vi "test Handle To Owned.vi"(8 "error in (no error)":errorcluster, 11 "TestCase in":refnum<class "Memory Manager Tests.lvclass">) -> (0 "error out":errorcluster, 3 "TestCase out":refnum<class "Memory Manager Tests.lvclass">)   [LabVIEW 2020, in "Memory Manager Tests.lvclass"]
uses:
  Memory Manager Tests.lvclass
  <vilib>/Utility/file.llb/Application Directory.vi
  <vilib>/Utility/libraryn.llb/Check if File or Folder Exists.vi
  <vilib>/addons/_JKI Toolkits/VI Tester/TestCase.llb/TestCase.lvclass
  C:/Program Files/National Instruments/LabVIEW 2024/vi.lib/addons/_JKI Toolkits/VI Tester/TestCase.llb/TestCase.lvclass
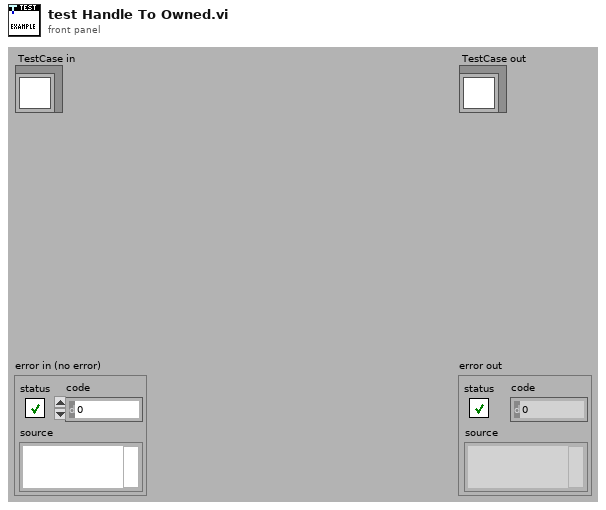
[diagram p1: front panel]
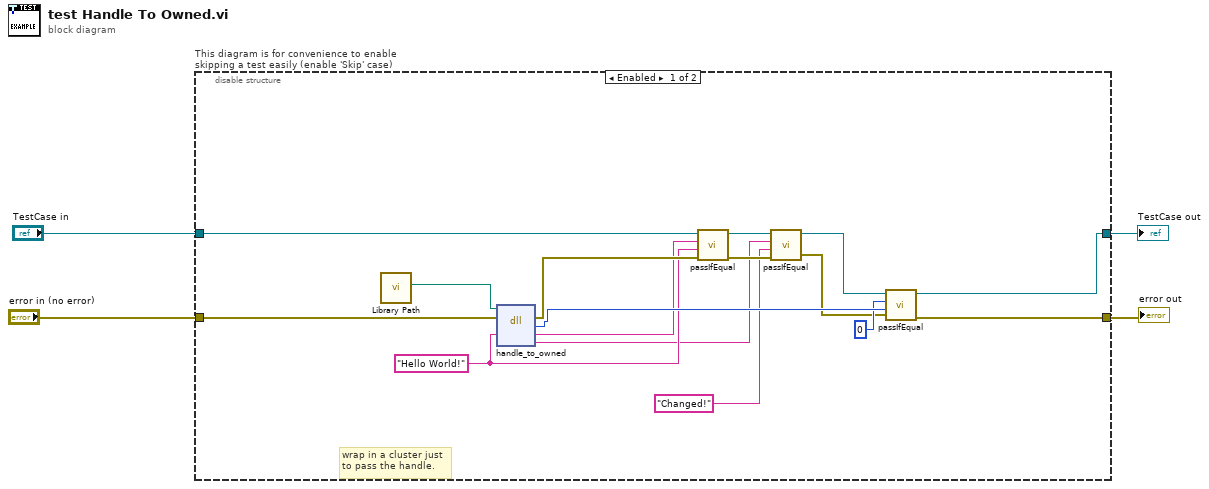
[diagram p0: block diagram]
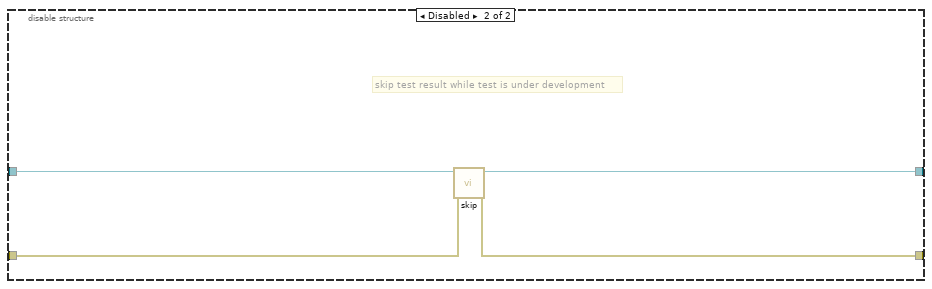
[diagram p2: hidden frame]
diagram:
  n1 = disable-structure "This diagram is for convenience to enable skipping a test easily (enable 'Skip' case)" shown="Enabled" {
    disable-tunnel: "TestCase in" -> [w20 w24]
    disable-tunnel: [w14 w22] -> w1
    disable-tunnel: [w15 w23] -> w3
    disable-tunnel: "error in (no error)" -> [w17 w21]
    frame Enabled {
      w8 = "Hello World!"
      # "wrap in a cluster just\nto pass the handle."
      n2 = call "Library Path.vi"() -> ("Library Path"=w18:path)  [unwired: 11 in]
      n3 = dll-call lib="C:/Users/JamesMcNally/Documents/RustInterop/Rust-LabVIEW-Interop/target/debug/labview_test_library.dll" fn="handle_to_owned"(path in=w18, error in=w17, "input"=w8) -> (error out=w16:errorcluster, "return type"=w13:i32, "input"=w7:string, "output"=w6:string)  [unwired: 2 in, 1 out]
      n4 = call-dynamic "passIfEqual.vi"("error in (no error)"=w16, "y"=w8, "x"=w7, "TestCase in"=w20) -> ("error out"=w19:errorcluster, "TestCase out"=w10:refnum<class "Memory Manager Tests.lvclass">)  [unwired: 6 in]
      n5 = call-dynamic "passIfEqual.vi"("error in (no error)"=w19, "y"="Changed!", "x"=w6, "TestCase in"=w10) -> ("error out"=w11:errorcluster, "TestCase out"=w9:refnum<class "Memory Manager Tests.lvclass">)  [unwired: 6 in]
      n6 = call-dynamic "passIfEqual.vi"("error in (no error)"=w11, "y"=w13, "x"=0 ("return type"), "TestCase in"=w9) -> ("error out"=w15:errorcluster, "TestCase out"=w14:refnum<class "Memory Manager Tests.lvclass">)  [unwired: 6 in]
    }
    frame Disabled {
      # "skip test result while test is under development"
      n7 = call <vilib>:"skip.vi"("error in (no error)"=w21, "TestCase in"=w24) -> ("error out"=w23:errorcluster, "TestCase out"=w22:refnum<class "Memory Manager Tests.lvclass">)  [unwired: 8 in]
    }
  }
  "error out" <- w3
  "TestCase out" <- w1
